vi "New Sensor.vi"(8 "Error In":errorcluster) -> (0 "Error Out":errorcluster, 2 "SensorName Out":string, 3 "Status":enum16{"OK", "Cancel"}(ring))   [LabVIEW 2019]
panel:
  in  "Cancel Button":bool
  in  "OK Button":bool
  in  "SensorName":string caption="Sensor Name:"
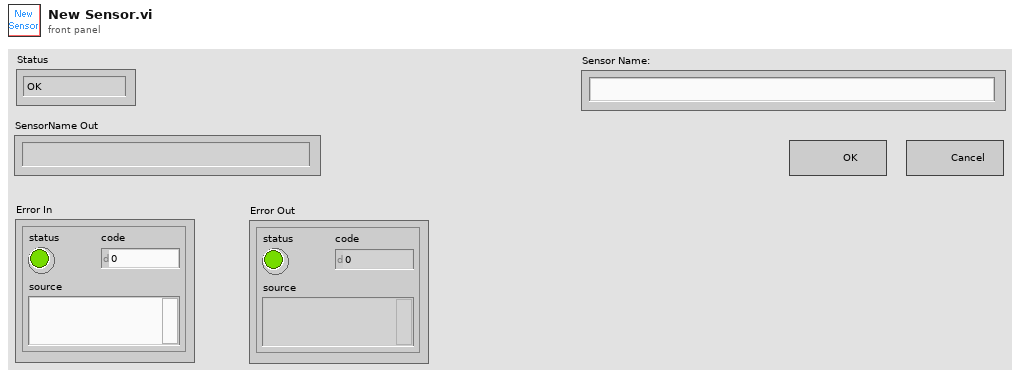
[diagram p1: front panel]
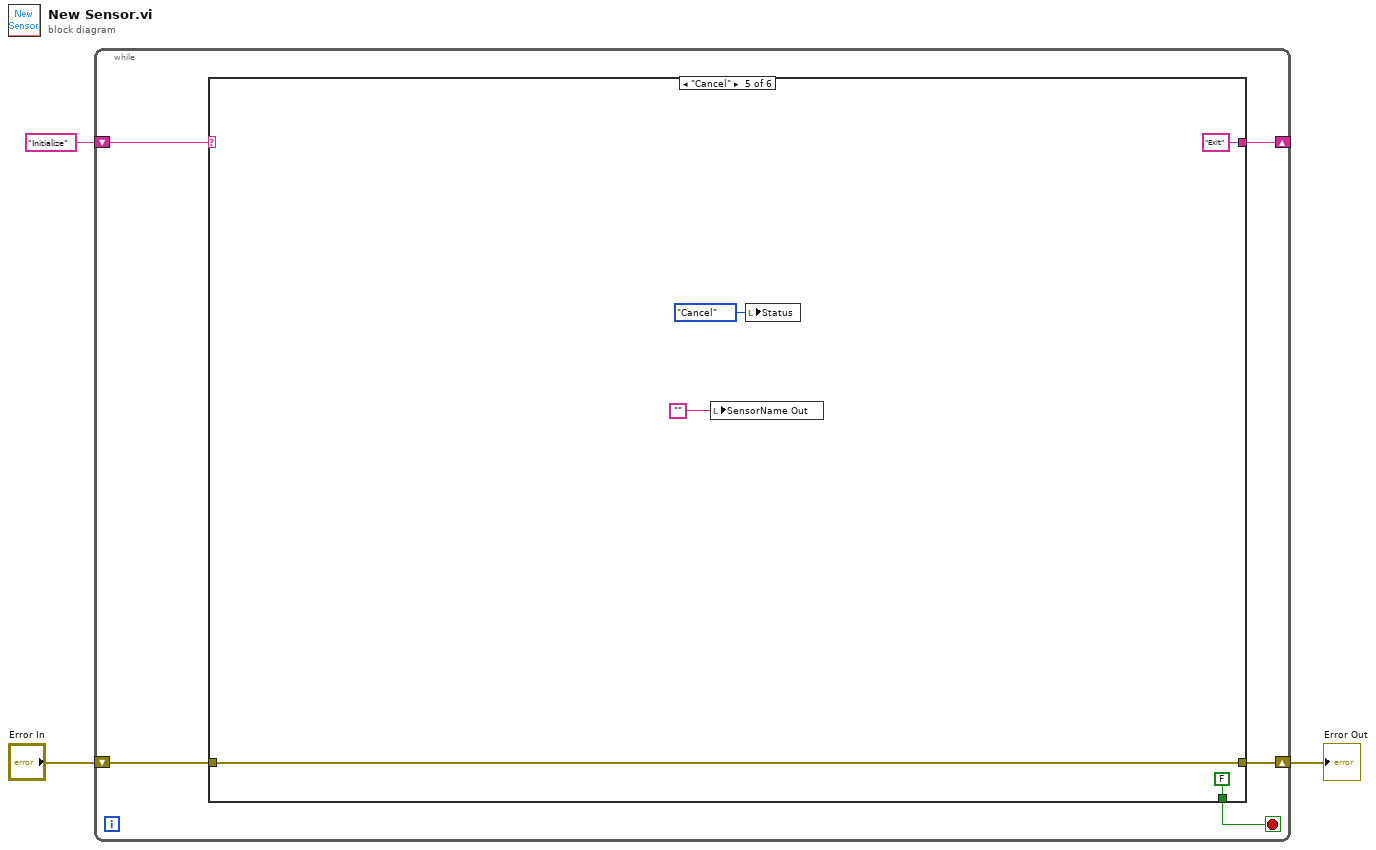
[diagram p0: block diagram]
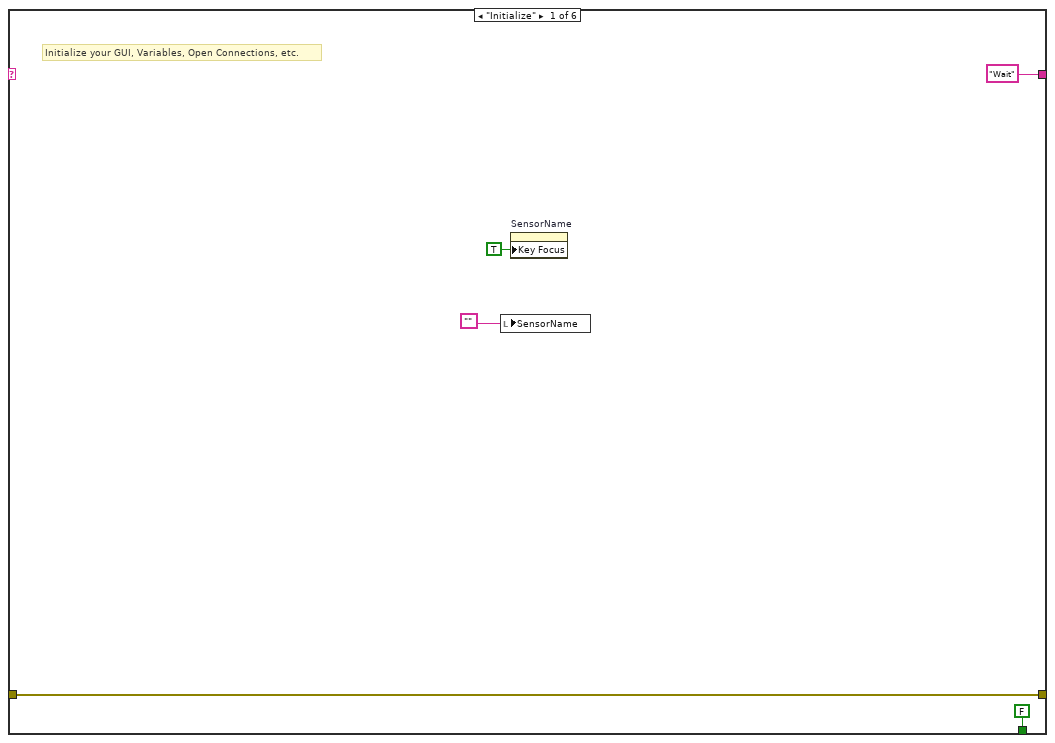
[diagram p2: hidden frame]
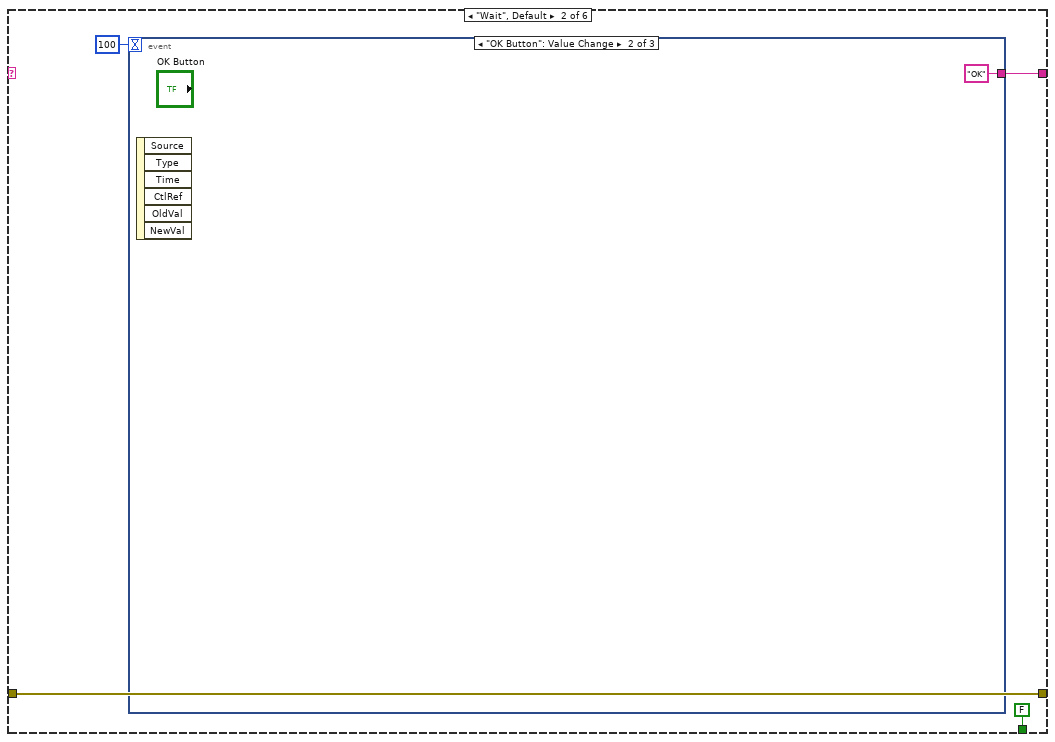
[diagram p3: hidden frame]
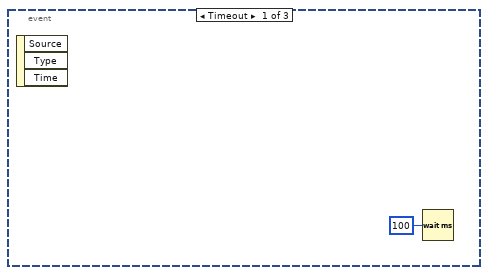
[diagram p4: hidden frame]
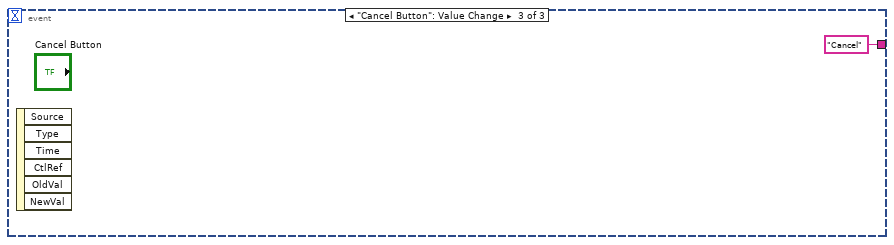
[diagram p5: hidden frame]
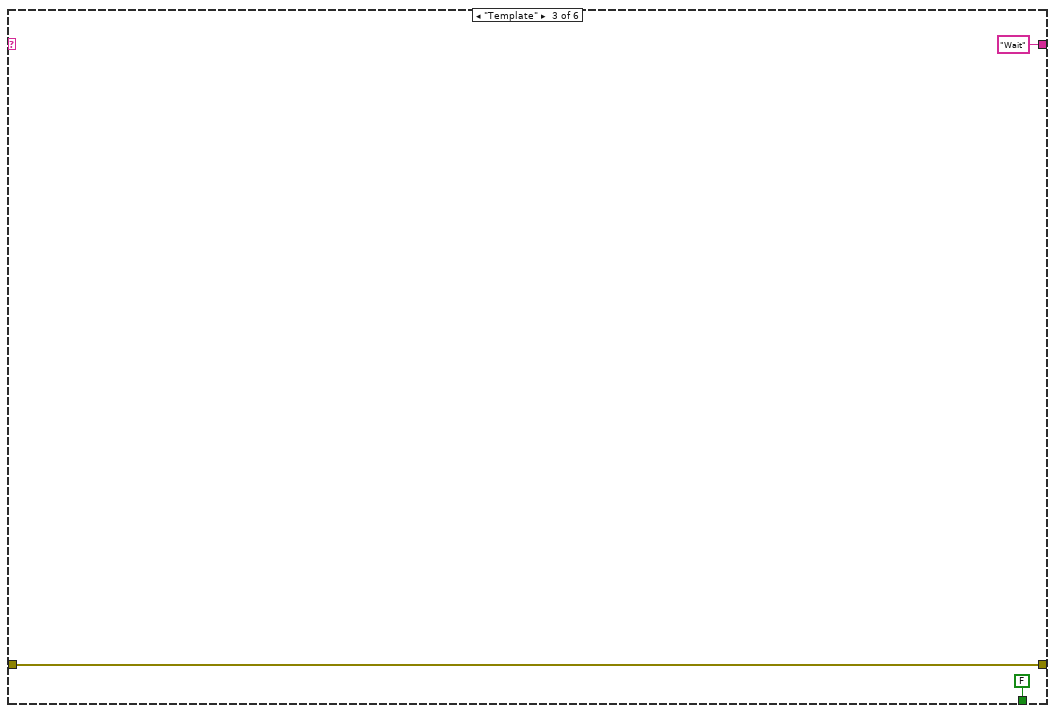
[diagram p6: hidden frame]
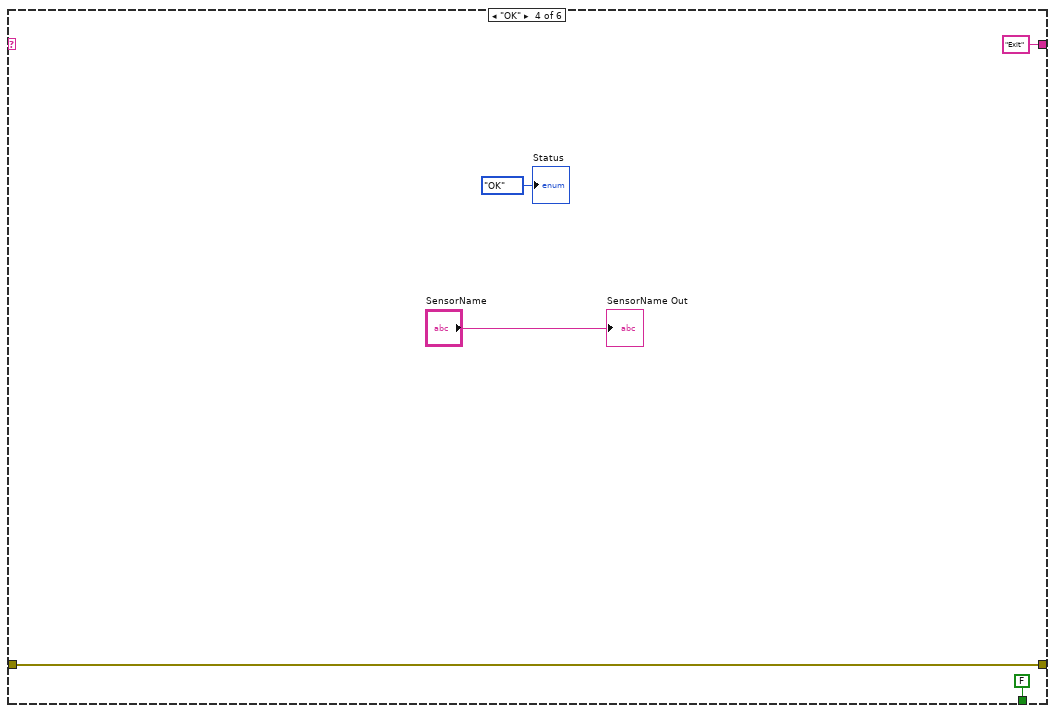
[diagram p7: hidden frame]
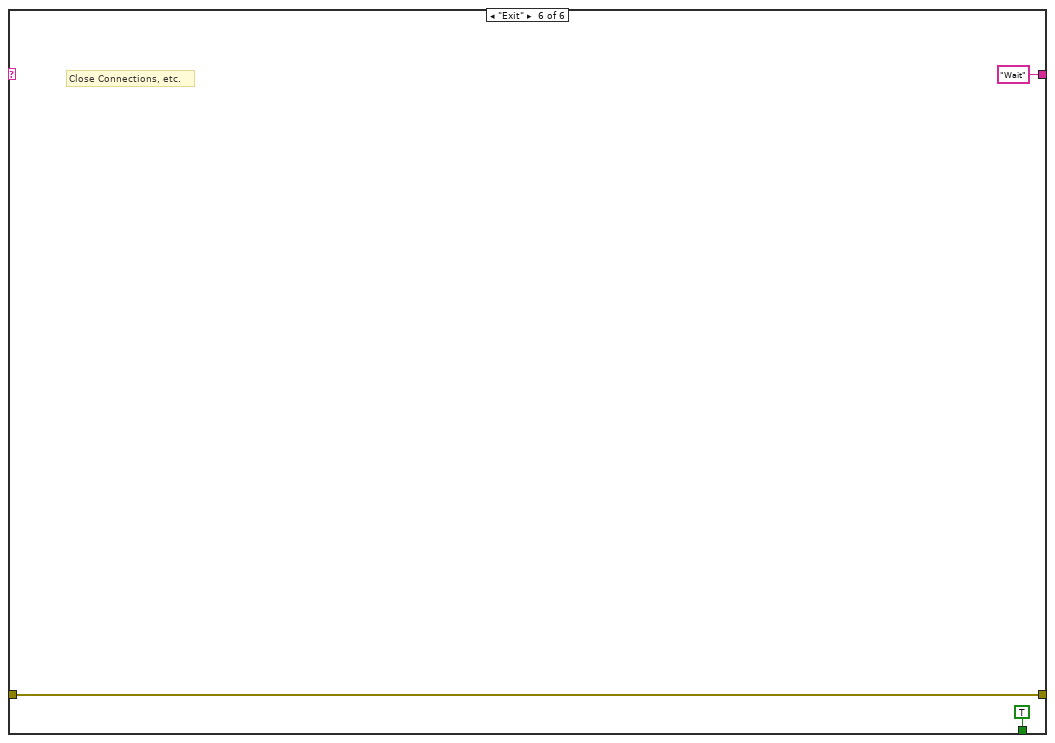
[diagram p8: hidden frame]
diagram:
  n1 = while {
    shift-right: [w7] -> _
    shift-left: "Initialize" -> [w8]
    shift-right: [w4] -> w1
    shift-left: "Error In" -> [w5]
    stop <- w6 stop-if-true
    n2 = case shown="\"Cancel\"" w8 {
      tunnel: ["Wait" w15 "Wait" "Exit" "Exit" "Wait"] -> w7
      tunnel: [FALSE FALSE FALSE FALSE FALSE TRUE] -> w6
      tunnel: w5 -> [w10 w14 w21 w25 w30 w34]
      tunnel: [w10 w14 w21 w25 w30 w34] -> w4
      frame "Initialize" {
        # "Initialize your GUI, Variables, Open Connections, etc."
        n3 = local write "SensorName"("") -> ()
        n4 = property on="SensorName" class="Str"("Key Focus"=TRUE) -> ()  [unwired: 2 in, 2 out]
      }
      frame "Wait", Default {
        n5 = event shown="[1] \"OK Button\": Value Change" {
          selector: _ -> [_ _ _]
          dyn-events: _ -> [_ _ _]
          timeout: 100 -> [_ _ _]
          tunnel: [_ "OK" "Cancel"] -> w15
          event Timeout {
            n6 = event-data() -> ()  [unwired: 1 in, 3 out]
            n7 = Wait (ms)(milliseconds to wait=u32 100) -> ()  [unwired: 1 out]
          }
          event "OK Button": Value Change {
            n8 = event-data() -> ()  [unwired: 1 in, 6 out]
          }
          event "Cancel Button": Value Change {
            n9 = event-data() -> ()  [unwired: 1 in, 6 out]
          }
        }
      }
      frame "Template" {
      }
      frame "OK" {
        "SensorName Out" <- "SensorName"
        "Status" <- enum16{"OK", "Cancel"}."OK" ("Status")
      }
      frame "Cancel" {
        n10 = local write "SensorName Out"("") -> ()
        n11 = local write "Status"(enum16{"OK", "Cancel"}."Cancel" ("Status")) -> ()
      }
      frame "Exit" {
        # "Close Connections, etc."
      }
    }
  }
  "Error Out" <- w1
